vi "_PluginLoader_Init.vi"(8 "error in (no error)":errorcluster, 10 "PluginsPath":path) -> (0 "error out":errorcluster, 3 "_PluginLoader out":refnum<class "_PluginLoader.lvclass">)   [LabVIEW 2014, in "_PluginLoader.lvclass"]
uses:
  _PluginLoader.lvclass
  _PluginLoader.lvclass/_PluginLoader.ctl
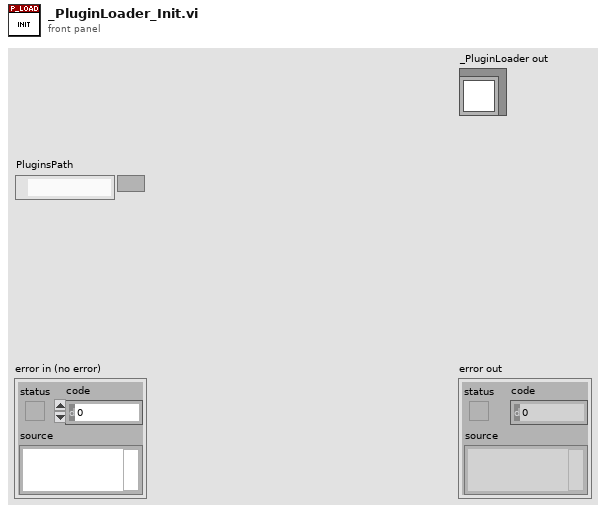
[diagram p1: front panel]
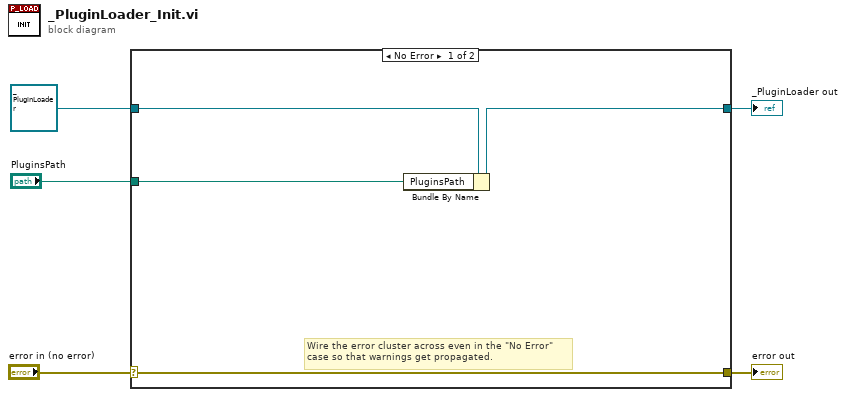
[diagram p0: block diagram]
diagram:
  n1 = case shown="No Error" "error in (no error)" {
    selector: "error in (no error)" -> [w8 w11]
    tunnel: [w8 w11] -> w4
    tunnel: [w7 w10] -> w2
    tunnel: refnum<class "_PluginLoader.lvclass"> refnum ("_PluginLoader in") -> [w9 w10]
    tunnel: "PluginsPath" -> [w6 _]
    frame No Error {
      # "Wire the error cluster across even in the \"No Error\"\ncase so that warnings get propagated."
      n2 = Bundle By Name(cluster=w9, "PluginsPath"=w6) -> (w7:refnum<class "_PluginLoader.lvclass">)
    }
    frame Error {
    }
  }
  "error out" <- w4
  "_PluginLoader out" <- w2
